vi "3.vi"(8 "error in (no error)":errorcluster, 11 "String":string) -> (0 "error in (no error) (dup)":errorcluster, 3 "The Count":string)   [LabVIEW 2017]
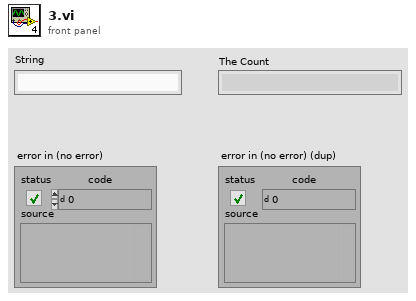
[diagram p1: front panel]
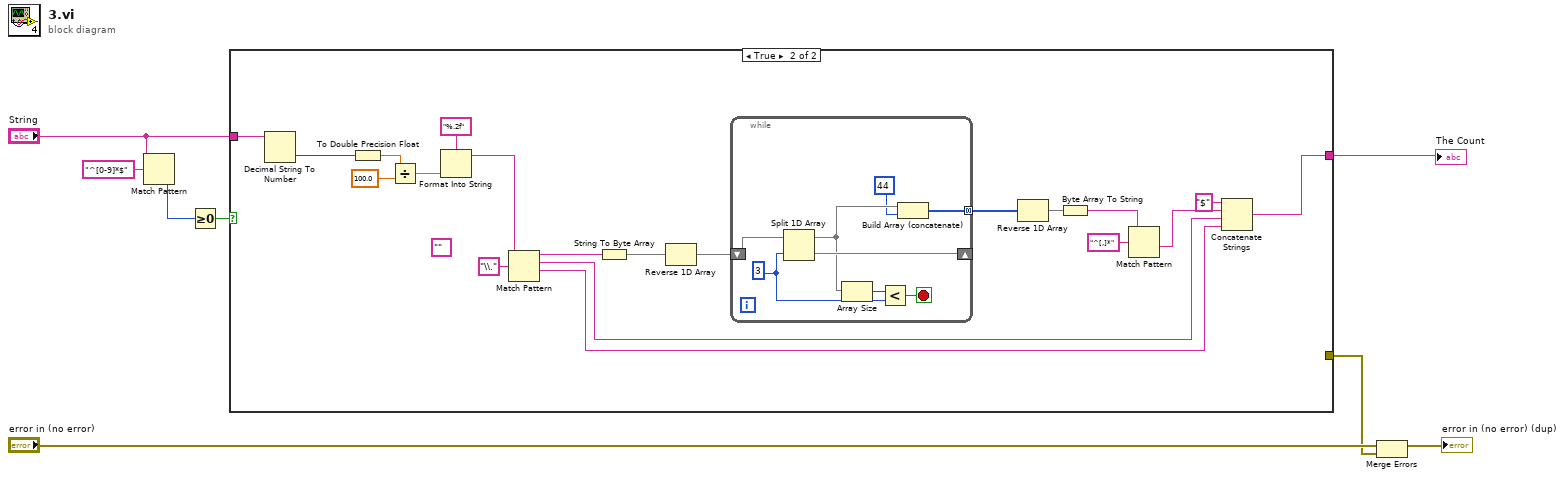
[diagram p0: block diagram]
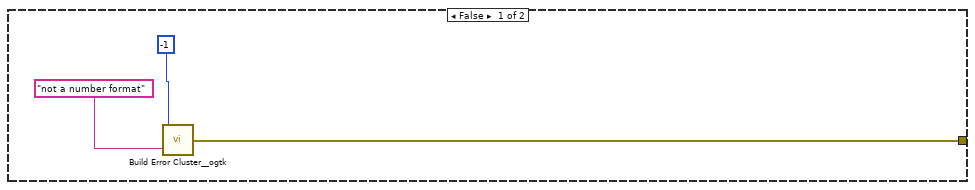
[diagram p2: hidden frame]
diagram:
  n1 = Match Pattern(string="String", regular expression="^[0-9]*$") -> (offset past match=w5:i32)  [unwired: 1 in, 3 out]
  n2 = Greater Or Equal To 0?(x=w5) -> (x >= 0?=w4:bool)
  n3 = case shown="True" w4 {
    tunnel: [_ w22] -> w7
    tunnel: [w9 _] -> w2
    tunnel: "String" -> [_ w31]
    frame False {
      n4 = call <userlib>:"Build Error Cluster__ogtk.vi"("String to Prepend to source (\"\")"="not a number format" ("String to Prepend to source (\"\")"), "code"=-1) -> ("error out"=w9:errorcluster)
    }
    frame True {
      (unwired) "" ("regular expression")
      n5 = Decimal String To Number(string=w31) -> (number=w30:i32)  [unwired: 2 in, 1 out]
      n6 = To Double Precision Float(number=w30) -> (double precision float=w29:dbl)
      n7 = Divide(x=w29, y=100.0) -> (x/y=w27:dbl)
      n8 = Format Into String(format string="%.2f", w27) -> (resulting string=w24:string)  [unwired: 2 in, 1 out]
      n9 = Match Pattern(string=w24, regular expression="\\.") -> (before substring=w23:string, match substring=w21:string, after substring=w20:string)  [unwired: 1 in, 1 out]
      n10 = String To Byte Array(string=w23) -> (unsigned byte array=w18:u8[])
      n11 = Reverse 1D Array(array=w18) -> (reversed array=w16:u8[])
      n12 = while {
        shift-right: [w38] -> _
        shift-left: w16 -> [w39]
        tunnel: [w37] -> w17 mode=concatenating
        stop <- w33 stop-if-true
        w34 = 3 ("index")
        n13 = Split 1D Array(array=w39, index=w34) -> (first subarray=w36:u8[], second subarray=w38:u8[])
        n14 = Array Size(array=w36) -> (size(s)=w35:i32)
        n15 = Less?(x=w35, y=w34) -> (x < y?=w33:bool)
        n16 = Build Array (concatenate)(w36, u8 44) -> (w37:u8[])
      }
      n17 = Reverse 1D Array(array=w17) -> (reversed array=w15:u8[])
      n18 = Byte Array To String(unsigned byte array=w15) -> (string=w13:string)
      n19 = Match Pattern(string=w13, regular expression="^[,]*") -> (after substring=w12:string)  [unwired: 1 in, 3 out]
      n20 = Concatenate Strings("$" ("string"), w12, w21, w20) -> (w22:string)
    }
  }
  "The Count" <- w7
  n21 = Merge Errors("error in (no error)", w2) -> (→"error in (no error) (dup)":errorcluster)
